vi "sgp4Calculator.vi"(9 "output cluster":T2, 10 "tsince":dbl) -> (0 "v":cdb[][](array[numeric]), 1 "r":cdb[][](array[numeric]), 2 "satrec":T1)   [LabVIEW 2015]
uses:
  <vilib>/imath/engines/lvmath/Plug In/_Char/NIMS_CH_character datatype.ctl
  <vilib>/imath/engines/lvmath2/RunTimeEngine/Managers/WorkSpace/UID Generator.vi
  <vilib>/imath/engines/lvmath2/RunTimeEngine/RunTimeType/NIMS_RunTimeType_From StrictType (excl LVString).vi
  <instcachedir>/0/NIMS_RunTimeType_From StrictType (excl LVString)_EB1C38A9BC5048DA9ABDA8F781E54D21.lvgen/NIMS_RunTimeType_From StrictType (excl LVString)_EB1C38A9BC5048DA9ABDA8F781E54D21_032.vi
  <instcachedir>/0/NIMS_RunTimeType_From StrictType (excl LVString)_EB1C38A9BC5048DA9ABDA8F781E54D21.lvgen/NIMS_RunTimeType_From StrictType (excl LVString)_EB1C38A9BC5048DA9ABDA8F781E54D21_031.vi
  <vilib>/imath/engines/lvmath/Plug In/_Char/NIMS_CH_String CV to Character 2D.vi
  <instcachedir>/0/NIMS_CH_String CV to Character 2D_EC8CCB3F0D074D66A728E5B1D55F815A.lvgen/NIMS_CH_String CV to Character 2D_EC8CCB3F0D074D66A728E5B1D55F815A_000.vi
  <instcachedir>/0/NIMS_RunTimeType_From StrictType (excl LVString)_EB1C38A9BC5048DA9ABDA8F781E54D21.lvgen/NIMS_RunTimeType_From StrictType (excl LVString)_EB1C38A9BC5048DA9ABDA8F781E54D21_001.vi
  <vilib>/imath/engines/lvmath2/RunTimeEngine/Struct/NIMS_StructSetField.vi
  <vilib>/imath/engines/lvmath2/RunTimeEngine/Struct/NIMS_StructGetField.vi
  <vilib>/imath/engines/lvmath2/RunTimeEngine/RunTimeType/NIMS_RunTimeType_To Numeric.vi
  <instcachedir>/0/NIMS_RunTimeType_To Numeric_B134FEC7BFC54ED5998F4CFD2EE98288.lvgen/NIMS_RunTimeType_To Numeric_B134FEC7BFC54ED5998F4CFD2EE98288_009.vi
  <instcachedir>/0/NIMS_RunTimeType_To Numeric_B134FEC7BFC54ED5998F4CFD2EE98288.lvgen/NIMS_RunTimeType_To Numeric_B134FEC7BFC54ED5998F4CFD2EE98288_008.vi
  <instcachedir>/0/NIMS_RunTimeType_From StrictType (excl LVString)_EB1C38A9BC5048DA9ABDA8F781E54D21.lvgen/NIMS_RunTimeType_From StrictType (excl LVString)_EB1C38A9BC5048DA9ABDA8F781E54D21_000.vi
  <vilib>/imath/engines/lvmath2/RunTimeEngine/LocalVariableDefStatement/MC_LocalVariableDefStatement_Display.vi
  <vilib>/imath/engines/lvmath2/RunTimeEngine/ArithmeticOperatorToken/NIMS_ArithmeticOperator_power(S).vi
  <instcachedir>/0/NIMS_ArithmeticOperator_power(S)_DFB67823F1414E5097C86E39787D8CA8.lvgen/NIMS_ArithmeticOperator_power(S)_DFB67823F1414E5097C86E39787D8CA8_014.vi
  <vilib>/imathl/engines/lvmath/Functions/Error Handling/Create Error.vi
  <instcachedir>/0/NIMS_ArithmeticOperator_power(S)_DFB67823F1414E5097C86E39787D8CA8.lvgen/NIMS_ArithmeticOperator_power(S)_DFB67823F1414E5097C86E39787D8CA8_009.vi
  <vilib>/imath/engines/lvmath2/RunTimeEngine/BuiltInFunctions/rem/NIMS_rem_no checks.vi
  <instcachedir>/0/NIMS_rem_no checks_948DC4F3B45040069021B8F54D02F312.lvgen/NIMS_rem_no checks_948DC4F3B45040069021B8F54D02F312_000.vi
  <vilib>/imath/engines/lvmath2/RunTimeSupport/NIMS_Complex To Real.vi
  <instcachedir>/0/NIMS_Complex To Real_01315F44AA8B4CE79FEF95AE999DC25E.lvgen/NIMS_Complex To Real_01315F44AA8B4CE79FEF95AE999DC25E_001.vi
  <vilib>/imath/engines/lvmath2/RunTimeEngine/BuiltInFunctions/abs/NIMS_abs(signed).vi
  <instcachedir>/0/NIMS_abs(signed)_C4FCB8E6058B49B797C7C8D53CA5F6EC.lvgen/NIMS_abs(signed)_C4FCB8E6058B49B797C7C8D53CA5F6EC_002.vi
  <vilib>/imath/engines/lvmath2/RunTimeEngine/CommandStatement/MC_CommandStatement_break.vi
  <vilib>/imath/engines/lvmath2/RunTimeEngine/BuiltInFunctions/sin/NIMS_sin(C).vi
  <instcachedir>/0/NIMS_sin(C)_93B37CF23FEA46B381CCAA607B2209DC.lvgen/NIMS_sin(C)_93B37CF23FEA46B381CCAA607B2209DC_001.vi
  <vilib>/imath/engines/lvmath2/RunTimeEngine/BuiltInFunctions/cos/NIMS_cos(C).vi
  <instcachedir>/0/NIMS_cos(C)_840A8FDA839D4E2AADB43697F53F61ED.lvgen/NIMS_cos(C)_840A8FDA839D4E2AADB43697F53F61ED_001.vi
  <vilib>/imath/engines/lvmath2/RunTimeEngine/CommandStatement/NIMS_CommandStatement_MaskErr.vi
  <vilib>/imath/engines/lvmath2/RunTimeEngine/VariableToken/NIMS_VariableToken_CondDefined.vi
  <instcachedir>/0/NIMS_VariableToken_CondDefined_FE30D0A1BFB24F098D41DEBABFE96BE1.lvgen/NIMS_VariableToken_CondDefined_FE30D0A1BFB24F098D41DEBABFE96BE1_003.vi
  <vilib>/imath/engines/lvmath2/RunTimeEngine/ErrorHandling/NIMS_Create Error From Enums.vi
  <vilib>/imath/engines/lvmath2/RunTimeEngine/BuiltInFunctions/atan2/NIMS_atan2.vi
  <instcachedir>/0/NIMS_atan2_A91AA4A7D42247EDBE8F76DB99AF04A4.lvgen/NIMS_atan2_A91AA4A7D42247EDBE8F76DB99AF04A4_000.vi
  <vilib>/imath/engines/lvmath/Plug In/_Char/RunTimeType/NIMS_CH_RunTimeType_To Character 2D.vi
  <vilib>/imath/engines/lvmath/Plug In/_Char/NIMS_CH_Character 2D to U8 2D.vi
  <vilib>/imath/engines/lvmath2/RunTimeEngine/IndexReplace/NIMS V(S)=S.vi
  <instcachedir>/0/NIMS V(S)=S_9916D32195284AEB9D40BA9A64F3B0C5.lvgen/NIMS V(S)=S_9916D32195284AEB9D40BA9A64F3B0C5_001.vi
  <vilib>/imath/engines/lvmath2/RunTimeEngine/Managers/SymbolTable/Clear UID.vi
  <vilib>/imath/engines/lvmath2/RunTimeEngine/NodeEndStatement/NIMS_NodeEndStatement_Output.vi
  <instcachedir>/0/NIMS_NodeEndStatement_Output_53EC0D466D134D7ABD903AC30B43404B.lvgen/NIMS_NodeEndStatement_Output_53EC0D466D134D7ABD903AC30B43404B_003.vi
  <vilib>/imath/engines/lvmath/Plug In/_Char/NIMS_CH_Character 2D to String 1D.vi
  <instcachedir>/0/NIMS_NodeEndStatement_Output_53EC0D466D134D7ABD903AC30B43404B.lvgen/NIMS_NodeEndStatement_Output_53EC0D466D134D7ABD903AC30B43404B_010.vi
  <vilib>/imath/engines/lvmath2/RunTimeEngine/ErrorHandling/NIMS_Finalize Error.vi
  <vilib>/imath/engines/lvmath2/RunTimeEngine/Managers/SymbolTable/NIMS_WorkSpace.lvlib
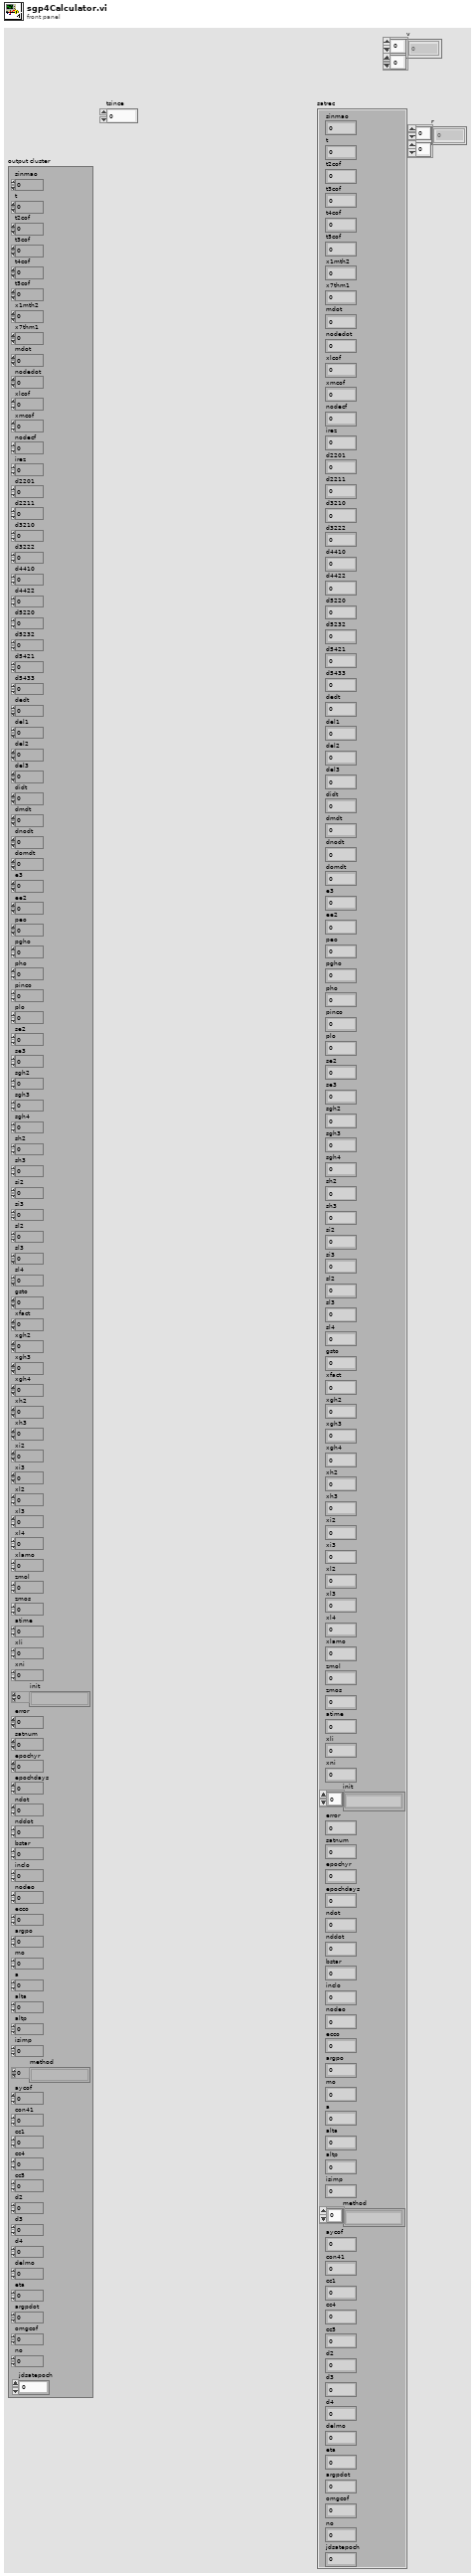
[diagram p1: front panel]
types:
  T1 = cluster{"sinmao":sgl, "t":dbl, "t2cof":sgl, "t3cof":sgl, "t4cof":sgl, "t5cof":sgl, "x1mth2":dbl, "x7thm1":dbl, "mdot":sgl, "nodedot":sgl, "xlcof":sgl, "xmcof":sgl, "nodecf":sgl, "irez":sgl, "d2201":sgl, "d2211":sgl, "d3210":sgl, "d3222":sgl, "d4410":sgl, "d4422":sgl, "d5220":sgl, "d5232":sgl, "d5421":sgl, "d5433":sgl, "dedt":sgl, "del1":sgl, "del2":sgl, "del3":sgl, "didt":sgl, "dmdt":sgl, "dnodt":sgl, "domdt":sgl, "e3":sgl, "ee2":sgl, "peo":sgl, "pgho":sgl, "pho":sgl, "pinco":sgl, "plo":sgl, "se2":sgl, "se3":sgl, "sgh2":sgl, "sgh3":sgl, "sgh4":sgl, "sh2":sgl, "sh3":sgl, "si2":sgl, "si3":sgl, "sl2":sgl, "sl3":sgl, "sl4":sgl, "gsto":sgl, "xfact":sgl, "xgh2":sgl, "xgh3":sgl, "xgh4":sgl, "xh2":sgl, "xh3":sgl, "xi2":sgl, "xi3":sgl, "xl2":sgl, "xl3":sgl, "xl4":sgl, "xlamo":sgl, "zmol":sgl, "zmos":sgl, "atime":sgl, "xli":sgl, "xni":sgl, "init":string[], "error":sgl, "satnum":sgl, "epochyr":sgl, "epochdays":dbl, "ndot":sgl, "nddot":sgl, "bstar":sgl, "inclo":sgl, "nodeo":sgl, "ecco":sgl, "argpo":sgl, "mo":sgl, "a":sgl, "alta":sgl, "altp":sgl, "isimp":sgl, "method":string[], "aycof":sgl, "con41":dbl, "cc1":sgl, "cc4":sgl, "cc5":sgl, "d2":sgl, "d3":sgl, "d4":sgl, "delmo":sgl, "eta":sgl, "argpdot":sgl, "omgcof":sgl, "no":sgl, "jdsatepoch":dbl}
  T2 = cluster{"sinmao":sgl, "t":sgl, "t2cof":sgl, "t3cof":sgl, "t4cof":sgl, "t5cof":sgl, "x1mth2":sgl, "x7thm1":sgl, "mdot":sgl, "nodedot":sgl, "xlcof":sgl, "xmcof":sgl, "nodecf":sgl, "irez":sgl, "d2201":sgl, "d2211":sgl, "d3210":sgl, "d3222":sgl, "d4410":sgl, "d4422":sgl, "d5220":sgl, "d5232":sgl, "d5421":sgl, "d5433":sgl, "dedt":sgl, "del1":sgl, "del2":sgl, "del3":sgl, "didt":sgl, "dmdt":sgl, "dnodt":sgl, "domdt":sgl, "e3":sgl, "ee2":sgl, "peo":sgl, "pgho":sgl, "pho":sgl, "pinco":sgl, "plo":sgl, "se2":sgl, "se3":sgl, "sgh2":sgl, "sgh3":sgl, "sgh4":sgl, "sh2":sgl, "sh3":sgl, "si2":sgl, "si3":sgl, "sl2":sgl, "sl3":sgl, "sl4":sgl, "gsto":sgl, "xfact":sgl, "xgh2":sgl, "xgh3":sgl, "xgh4":sgl, "xh2":sgl, "xh3":sgl, "xi2":sgl, "xi3":sgl, "xl2":sgl, "xl3":sgl, "xl4":sgl, "xlamo":sgl, "zmol":sgl, "zmos":sgl, "atime":sgl, "xli":sgl, "xni":sgl, "init":string[], "error":sgl, "satnum":sgl, "epochyr":sgl, "epochdays":dbl, "ndot":sgl, "nddot":sgl, "bstar":sgl, "inclo":sgl, "nodeo":sgl, "ecco":sgl, "argpo":sgl, "mo":sgl, "a":sgl, "alta":sgl, "altp":sgl, "isimp":sgl, "method":string[], "aycof":sgl, "con41":sgl, "cc1":sgl, "cc4":sgl, "cc5":sgl, "d2":sgl, "d3":sgl, "d4":sgl, "delmo":sgl, "eta":sgl, "argpdot":sgl, "omgcof":sgl, "no":sgl, "jdsatepoch":dbl}
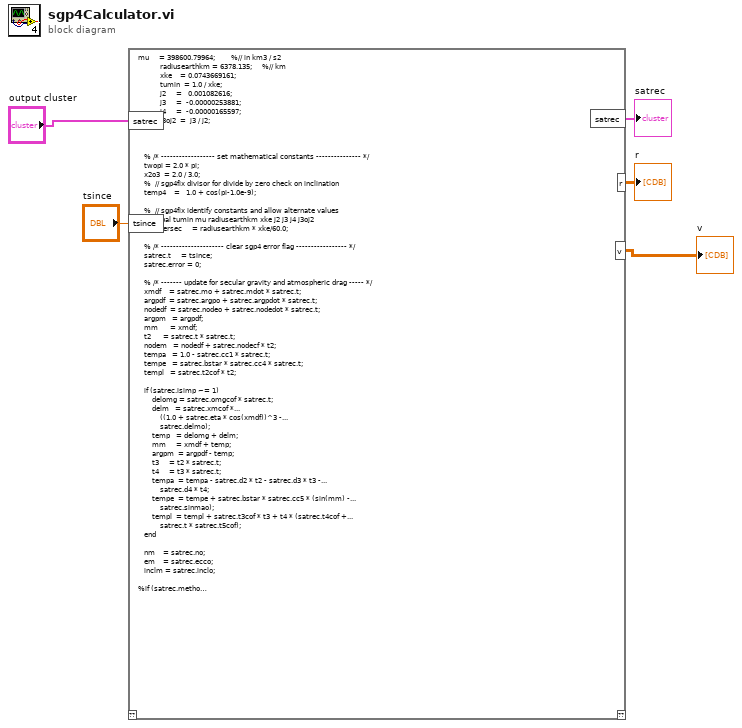
[diagram p0: block diagram]
diagram:
  n1 = mathscript code="mu     = 398600.79964;        %// in km3 / s2\n           radiusearthkm = 6378.135;     %// km\n           xke    = 0.0743669161;\n           tumin  = 1.0 / xke;\n           j2     =   0.001082616;\n           j3     =  -0.00000253881;\n           j4     =  -0.00000165597;\n           j3oj2  =  j3 / j2;\n\n\n\n   % /* ------------------ set mathematical constants --------------- */\n   twopi = 2.0 * pi;\n   x2o3  = 2.0 / 3.0;\n   %  // sgp4fix divisor for divide by zero check on inclination\n   temp4    =   1.0 + cos(pi-1.0e-9);\n\n   %  // sgp4fix identify constants and allow alternate values\n   %global tumin mu radiusearthkm xke j2 j3 j4 j3oj2  \n   vkmpersec     = radiusearthkm * xke/60.0;\n   \n   % /* --------------------- clear sgp4 error flag ----------------- */\n   satrec.t     = tsince;\n   satrec.error = 0;\n\n   % /* ------- update for secular gravity and atmospheric drag ----- */\n   xmdf    = satrec.mo + satrec.mdot * satrec.t;\n   argpdf  = satrec.argpo + satrec.argpdot * satrec.t;\n   nodedf  = satrec.nodeo + satrec.nodedot * satrec.t;\n   argpm   = argpdf;\n   mm      = xmdf;\n   t2      = satrec.t * satrec.t;\n   nodem   = nodedf + satrec.nodecf * t2;\n   tempa   = 1.0 - satrec.cc1 * satrec.t;\n   tempe   = satrec.bstar * satrec.cc4 * satrec.t;\n   templ   = satrec.t2cof * t2;\n\n   if (satrec.isimp ~= 1)\n       delomg = satrec.omgcof * satrec.t;\n       delm   = satrec.xmcof *...\n           ((1.0 + satrec.eta * cos(xmdf))^3 -...\n           satrec.delmo);\n       temp   = delomg + delm;\n       mm     = xmdf + temp;\n       argpm  = argpdf - temp;\n       t3     = t2 * satrec.t;\n       t4     = t3 * satrec.t;\n       tempa  = tempa - satrec.d2 * t2 - satrec.d3 * t3 -...\n           satrec.d4 * t4;\n       tempe  = tempe + satrec.bstar * satrec.cc5 * (sin(mm) -...\n           satrec.sinmao);\n       templ  = templ + satrec.t3cof * t3 + t4 * (satrec.t4cof +...\n           satrec.t * satrec.t5cof);\n   end\n\n   nm    = satrec.no;\n   em    = satrec.ecco;\n   inclm = satrec.inclo;\n   \n%if (satrec.method == 'd')\n       %tc = satrec.t;\n       %[satrec.atime,em,argpm,inclm,satrec.xli,mm,...\n         %  satrec.xni,nodem,dndt,nm] = dspace(...\n         %  satrec.d2201,satrec.d2211,satrec.d3210,...\n          % satrec.d3222,satrec.d4410,satrec.d4422,...\n          % satrec.d5220,satrec.d5232,satrec.d5421,...\n          % satrec.d5433,satrec.dedt,satrec.del1,...\n          % satrec.del2,satrec.del3,satrec.didt,...\n          % satrec.dmdt,satrec.dnodt,satrec.domdt,...\n          % satrec.irez,satrec.argpo,satrec.argpdot,satrec.t,...\n          % tc,satrec.gsto,satrec.xfact,satrec.xlamo,satrec.no,...\n          % satrec.atime,em,argpm,inclm,satrec.xli,mm,...\n          % satrec.xni,nodem,nm);\n  % end % // if method = d\n\n   if (nm <= 0.0)\n%       fprintf(1,'# error nm %f\\n', nm);\n       satrec.error = 2;\n\n\t\n   end\n\n%xke=1;\n%nm=1;\n   am = xke/nm\n   am=am^x2o3\n\tam=am* tempa * tempa;\n   nm = xke / am^1.5;\n   em = em - tempe;\n\n   % // fix tolerance for error recognition\n   if ((em >= 1.0) || (em < -0.001) || (am < 0.95))\n%       fprintf(1,'# error em %f\\n', em);\n       satrec.error = 1;\n   end\n   if (em < 0.0)\n       em  = 1.0e-6;\n   end\n   mm     = mm + satrec.no * templ;\n   xlm    = mm + argpm + nodem;\n   emsq   = em * em;\n   temp   = 1.0 - emsq;\n   nodem  = rem(nodem, twopi);\n   argpm  = rem(argpm, twopi);\n   xlm    = rem(xlm, twopi);\n   mm     = rem(xlm - argpm - nodem, twopi);\n\n   % /* ----------------- compute extra mean quantities ------------- */\n   sinim = sin(inclm);\n   cosim = cos(inclm);\n\n   % /* -------------------- add lunar-solar periodics -------------- */\n   ep     = em;\n   xincp  = inclm;\n   argpp  = argpm;\n   nodep  = nodem;\n   mp     = mm;\n   sinip  = sinim;\n   cosip  = cosim;\n\n\n%%%\n\n\n\n   % /* -------------------- long period periodics ------------------ */\n \n%%%%\n\n\n\n   axnl = ep * cos(argpp);\n   temp = 1.0 / (am * (1.0 - ep * ep));\n   aynl = ep* sin(argpp) + temp * satrec.aycof;\n   xl   = mp + argpp + nodep + temp * satrec.xlcof * axnl;\n\n   % /* --------------------- solve kepler's equation --------------- */\n   u    = rem(xl - nodep, twopi);\n   eo1  = u;\n   tem5 = 9999.9;\n   ktr = 1;\n   % //   sgp4fix for kepler iteration\n   % //   the following iteration needs better limits on corrections\n   while (( abs(tem5) >= 1.0e-12) && (ktr <= 10) )\n       sineo1 = sin(eo1);\n       coseo1 = cos(eo1);\n       tem5   = 1.0 - coseo1 * axnl - sineo1 * aynl;\n       tem5   = (u - aynl * coseo1 + axnl * sineo1 - eo1) / tem5;\n       if(abs(tem5) >= 0.95)\n           if tem5 > 0.0\n               tem5 = 0.95;\n           else\n               tem5 = -0.95;\n           end\n       end\n       eo1    = eo1 + tem5;\n       ktr = ktr + 1;\n   end\n\n   % /* ------------- short period preliminary quantities ----------- */\n   ecose = axnl*coseo1 + aynl*sineo1;\n   esine = axnl*sineo1 - aynl*coseo1;\n   el2   = axnl*axnl + aynl*aynl;\n   pl    = am*(1.0-el2);\n   if (pl < 0.0)\n%       fprintf(1,'# error pl %f\\n', pl);\n       satrec.error = 4;\n       r = [0;0;0];\n       v = [0;0;0];\n   else\n       rl     = am * (1.0 - ecose);\n       rdotl  = sqrt(am) * esine/rl;\n       rvdotl = sqrt(pl) / rl;\n       betal  = sqrt(1.0 - el2);\n       temp   = esine / (1.0 + betal);\n       sinu   = am / rl * (sineo1 - aynl - axnl * temp);\n       cosu   = am / rl * (coseo1 - axnl + aynl * temp);\n       su     = atan2(sinu, cosu);\n       sin2u  = (cosu + cosu) * sinu;\n       cos2u  = 1.0 - 2.0 * sinu * sinu;\n       temp   = 1.0 / pl;\n       temp1  = 0.5 * j2 * temp;\n       temp2  = temp1 * temp;\n\n       % /* -------------- update for short period periodics ------------ */\n       if (satrec.method == 'd')\n           cosisq                 = cosip * cosip;\n           satrec.con41  = 3.0*cosisq - 1.0;\n           satrec.x1mth2 = 1.0 - cosisq;\n           satrec.x7thm1 = 7.0*cosisq - 1.0;\n       end\n       mrt   = rl * (1.0 - 1.5 * temp2 * betal * satrec.con41) +...\n           0.5 * temp1 * satrec.x1mth2 * cos2u;\n       su    = su - 0.25 * temp2 * satrec.x7thm1 * sin2u;\n       xnode = nodep + 1.5 * temp2 * cosip * sin2u;\n       xinc  = xincp + 1.5 * temp2 * cosip * sinip * cos2u;\n       mvt   = rdotl - nm * temp1 * satrec.x1mth2 * sin2u / xke;\n       rvdot = rvdotl + nm * temp1 * (satrec.x1mth2 * cos2u +...\n           1.5 * satrec.con41) / xke;\n\n       % /* --------------------- orientation vectors ------------------- */\n       sinsu =  sin(su);\n       cossu =  cos(su);\n       snod  =  sin(xnode);\n       cnod  =  cos(xnode);\n       sini  =  sin(xinc);\n       cosi  =  cos(xinc);\n       xmx   = -snod * cosi;\n       xmy   =  cnod * cosi;\n       ux    =  xmx * sinsu + cnod * cossu;\n       uy    =  xmy * sinsu + snod * cossu;\n       uz    =  sini * sinsu;\n       vx    =  xmx * cossu - cnod * sinsu;\n       vy    =  xmy * cossu - snod * sinsu;\n       vz    =  sini * cossu;\n\n       % /* --------- position and velocity (in km and km/sec) ---------- */\n       r(1) = (mrt * ux)* radiusearthkm;\n       r(2) = (mrt * uy)* radiusearthkm;\n       r(3) = (mrt * uz)* radiusearthkm;\n       v(1) = (mvt * ux + rvdot * vx) * vkmpersec;\n       v(2) = (mvt * uy + rvdot * vy) * vkmpersec;\n       v(3) = (mvt * uz + rvdot * vz) * vkmpersec;\n   end % // if pl > 0\n\n       % // sgp4fix for decaying satellites\n        if (mrt < 1.0)\n   %         printf(\"# decay condition %11.6f \\n\",mrt);\n            satrec.error = 6;\n        end"("satrec"="output cluster", "tsince"="tsince") -> ("satrec"=→"satrec":T1, "r"=→"r":cdb[][], "v"=→"v":cdb[][])  [unwired: 1 in, 1 out]
